vi "LabviewProject_Nabors.vi"() -> ()   [LabVIEW 2017]
panel:
  out "RMS":dbl
  out "Minimum":dbl
  out "Maximum":dbl
  out "Arithmetic Mean":dbl
  out "Frequency":dbl format="%#_4g"
  out "Amplitude":dbl format="%#_4g"
  out "Period":dbl format="%#_4g"
  in  "Duty Cycle (%)":dbl(knob)=50.0 scale=0.0..100.0
  in  "Noise":enum16{"None", "Gaussian", "Uniform"}(ring)
  in  "Signal Type":T1(ring)
  in  "Amplitude":dbl(knob)=1.0 scale=0.0..10.0
  in  "Frequency":dbl(knob)=10.1 scale=0.0..20.0
  in  "Offset":dbl(knob) scale=-10.0..10.0 scale format="%#_10g"
  in  "stop":bool
  in  "Tab Control":enum32{"AFG", "FFT"}(tab)
  out "AFG Display":dynamicdata(graph) caption="Sine"
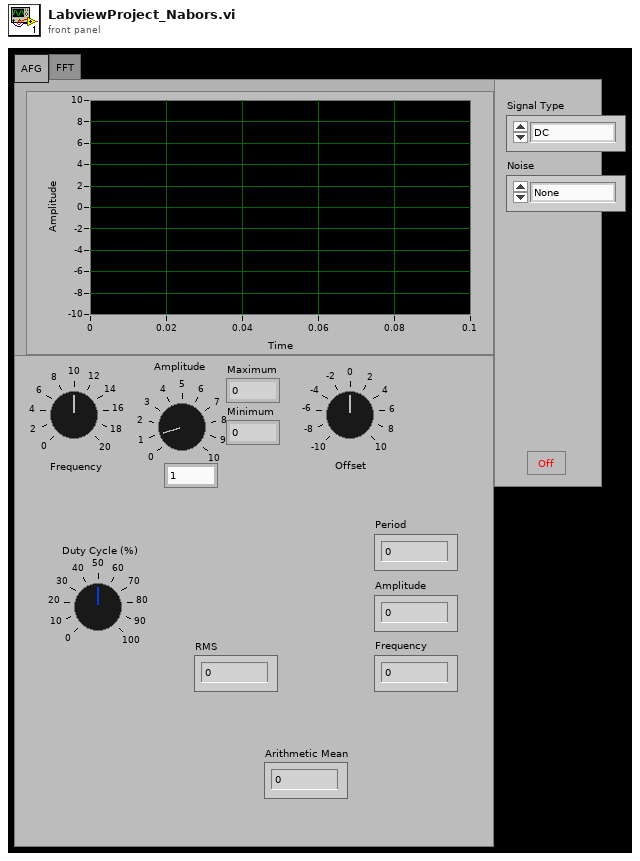
[diagram p1: front panel]
types:
  T1 = enum16{"DC", "Sine", "Square", "Sawtooth", "Triangular"}
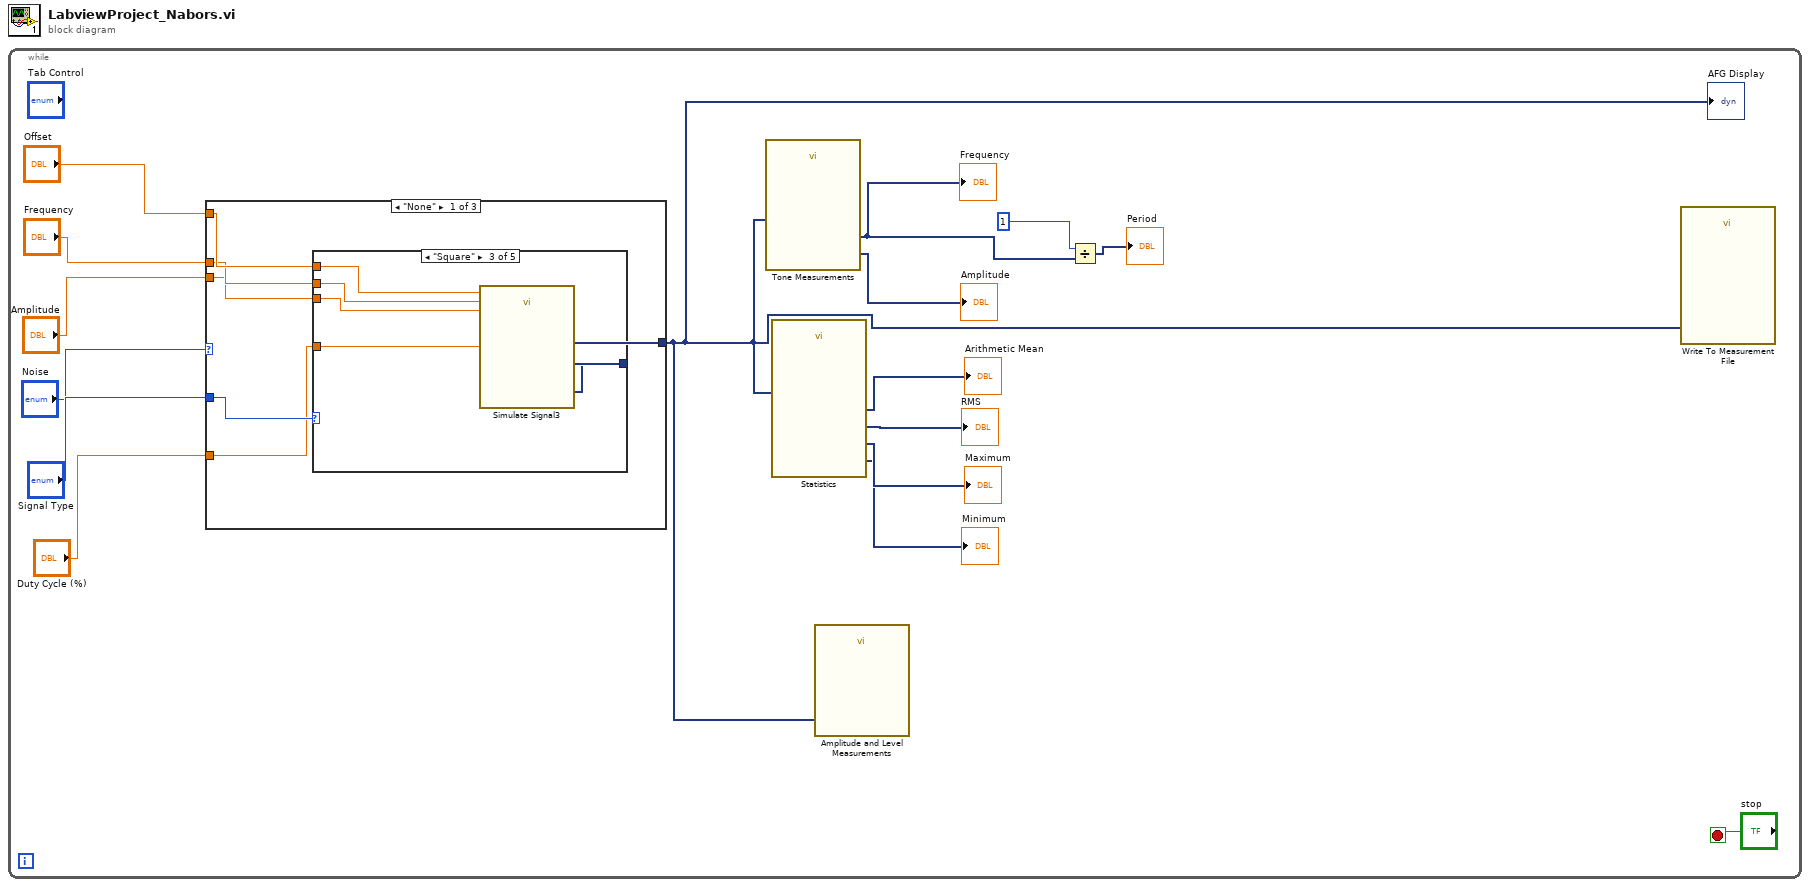
[diagram p0: block diagram]
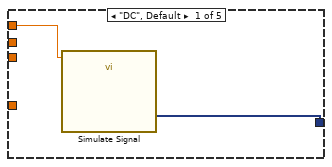
[diagram p2: hidden frame]
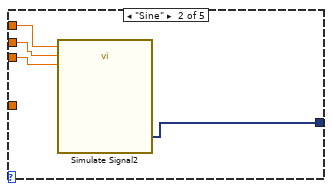
[diagram p3: hidden frame]
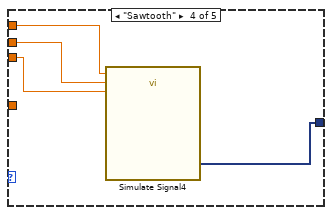
[diagram p4: hidden frame]
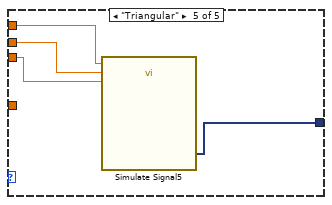
[diagram p5: hidden frame]
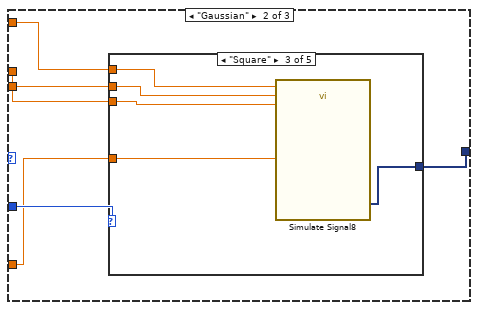
[diagram p6: hidden frame]
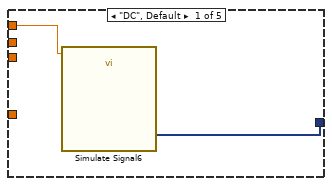
[diagram p7: hidden frame]
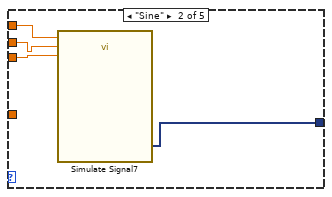
[diagram p8: hidden frame]
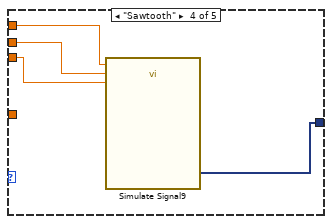
[diagram p9: hidden frame]
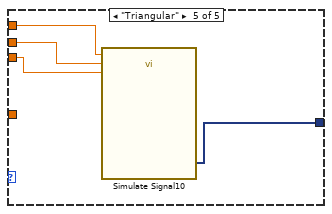
[diagram p10: hidden frame]
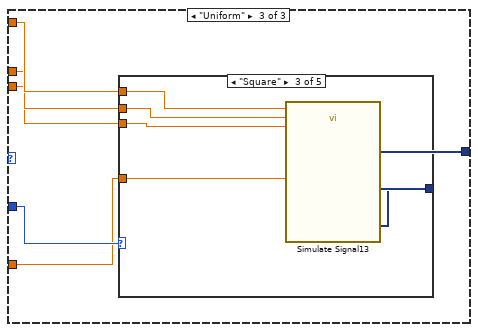
[diagram p11: hidden frame]
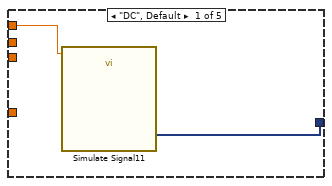
[diagram p12: hidden frame]
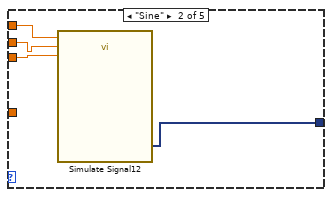
[diagram p13: hidden frame]
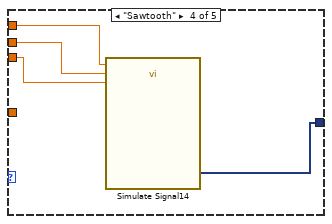
[diagram p14: hidden frame]
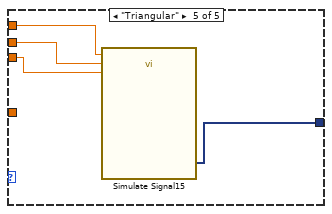
[diagram p15: hidden frame]
diagram:
  n1 = while {
    stop <- "stop" stop-if-true
    n2 = case shown="\"None\"" "Noise" {
      tunnel: "Signal Type" -> [w22 w43 w68]
      tunnel: "Offset" -> [w21 w44 w72]
      tunnel: "Frequency" -> [w20 w45 w71]
      tunnel: "Amplitude" -> [w19 w46 w70]
      tunnel: [w18 w47 w69] -> w1
      tunnel: "Duty Cycle (%)" -> [w17 w42 w67]
      frame "None" {
        n3 = case shown="\"Square\"" w22 {
          tunnel: w21 -> [w24 w28 w33 w37 w40]
          tunnel: w20 -> [_ w27 w32 w36 w39]
          tunnel: w19 -> [_ w26 w31 w35 w38]
          tunnel: [w23 w25 w30 w34 w41] -> w18
          tunnel: w17 -> [_ _ w29 _ _]
          frame "DC", Default {
            n4 = call "Simulate Signal"("Offset"=w24) -> ("DC"=w23:dynamicdata)  [unwired: 13 in, 1 out]
          }
          frame "Sine" {
            n5 = call "Simulate Signal2"("Offset"=w28, "Frequency"=w27, "Amplitude"=w26) -> ("Sine"=w25:dynamicdata)  [unwired: 11 in, 1 out]
          }
          frame "Square" {
            n6 = call "Simulate Signal3"("Offset"=w33, "Duty Cycle (%)"=w29, "Frequency"=w32, "Amplitude"=w31) -> ("Square"=w30:dynamicdata)  [unwired: 10 in, 1 out]
          }
          frame "Sawtooth" {
            n7 = call "Simulate Signal4"("Offset"=w37, "Frequency"=w36, "Amplitude"=w35) -> ("Sawtooth"=w34:dynamicdata)  [unwired: 11 in, 1 out]
          }
          frame "Triangular" {
            n8 = call "Simulate Signal5"("Offset"=w40, "Frequency"=w39, "Amplitude"=w38) -> ("Triangle"=w41:dynamicdata)  [unwired: 11 in, 1 out]
          }
        }
      }
      frame "Gaussian" {
        n9 = case shown="\"Square\"" w43 {
          tunnel: w44 -> [w49 w53 w58 w62 w65]
          tunnel: w45 -> [_ w52 w57 w61 w64]
          tunnel: w46 -> [_ w51 w56 w60 w63]
          tunnel: [w48 w50 w55 w59 w66] -> w47
          tunnel: w42 -> [_ _ w54 _ _]
          frame "DC", Default {
            n10 = call "Simulate Signal6"("Offset"=w49) -> ("DC with Gaussian Noise"=w48:dynamicdata)  [unwired: 13 in, 1 out]
          }
          frame "Sine" {
            n11 = call "Simulate Signal7"("Offset"=w53, "Frequency"=w52, "Amplitude"=w51) -> ("Sine with Gaussian Noise"=w50:dynamicdata)  [unwired: 11 in, 1 out]
          }
          frame "Square" {
            n12 = call "Simulate Signal8"("Offset"=w58, "Duty Cycle (%)"=w54, "Frequency"=w57, "Amplitude"=w56) -> ("Square with Gaussian Noise"=w55:dynamicdata)  [unwired: 10 in, 1 out]
          }
          frame "Sawtooth" {
            n13 = call "Simulate Signal9"("Offset"=w62, "Frequency"=w61, "Amplitude"=w60) -> ("Sawtooth with Gaussian Noise"=w59:dynamicdata)  [unwired: 11 in, 1 out]
          }
          frame "Triangular" {
            n14 = call "Simulate Signal10"("Offset"=w65, "Frequency"=w64, "Amplitude"=w63) -> ("Triangle with Gaussian Noise"=w66:dynamicdata)  [unwired: 11 in, 1 out]
          }
        }
      }
      frame "Uniform" {
        n15 = case shown="\"Square\"" w68 {
          tunnel: w72 -> [w74 w78 w83 w87 w90]
          tunnel: w71 -> [_ w77 w82 w86 w89]
          tunnel: w70 -> [_ w76 w81 w85 w88]
          tunnel: [w73 w75 w80 w84 w91] -> w69
          tunnel: w67 -> [_ _ w79 _ _]
          frame "DC", Default {
            n16 = call "Simulate Signal11"("Offset"=w74) -> ("DC with Uniform Noise"=w73:dynamicdata)  [unwired: 13 in, 1 out]
          }
          frame "Sine" {
            n17 = call "Simulate Signal12"("Offset"=w78, "Frequency"=w77, "Amplitude"=w76) -> ("Sine with Uniform Noise"=w75:dynamicdata)  [unwired: 11 in, 1 out]
          }
          frame "Square" {
            n18 = call "Simulate Signal13"("Offset"=w83, "Duty Cycle (%)"=w79, "Frequency"=w82, "Amplitude"=w81) -> ("Square with Uniform Noise"=w80:dynamicdata)  [unwired: 10 in, 1 out]
          }
          frame "Sawtooth" {
            n19 = call "Simulate Signal14"("Offset"=w87, "Frequency"=w86, "Amplitude"=w85) -> ("Sawtooth with Uniform Noise"=w84:dynamicdata)  [unwired: 11 in, 1 out]
          }
          frame "Triangular" {
            n20 = call "Simulate Signal15"("Offset"=w90, "Frequency"=w89, "Amplitude"=w88) -> ("Triangle with Uniform Noise"=w91:dynamicdata)  [unwired: 11 in, 1 out]
          }
        }
      }
    }
    "AFG Display" <- w1
    n21 = call "Tone Measurements"("Signals"=w1) -> ("Frequency"=w6:dynamicdata, "Amplitude"=→"Amplitude":dynamicdata)  [unwired: 8 in, 1 out]
    "Frequency" <- w6
    n22 = call "Statistics"("Signals"=w1) -> ("RMS"=→"RMS":dynamicdata, "Arithmetic Mean"=→"Arithmetic Mean":dynamicdata, "Minimum"=→"Minimum":dynamicdata, "Maximum"=→"Maximum":dynamicdata)  [unwired: 22 in, 1 out]
    n23 = call "Amplitude and Level Measurements"("Signals"=w1) -> ()  [unwired: 14 in, 1 out]
    n24 = Divide(x=1, y=w6) -> (x/y=→"Period":dynamicdata)
    n25 = call "Write To Measurement File"("Signals"=w1) -> ()  [unwired: 16 in, 3 out]
  }
